vi "SVT Integration.vi"   [LabVIEW 2017]
doc: "Converts acceleration to velocity or displacement. You can use this polymorphic VI to integrate signals for a single channel or for N channels. The data type you wire to the <B>scaled signal [EU]</B> input determines the polymorphic instance to use."
uses:
  <vilib>/addons/Sound and Vibration/svt_Integration/SoundVib_Integration.lvlib
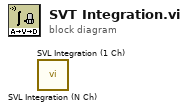
[diagram p0: block diagram]
diagram:
  n1 = call <vilib>:"SVL Integration (N Ch).vi"() -> ()  [unwired: 9 in, 3 out]
  n2 = call <vilib>:"SVL Integration (1 Ch).vi"() -> ()  [unwired: 9 in, 3 out]
